vi "CRYGet Selected Rows.vi"(10 "Right Clicked Row":i32=-1, 11 "Tree Ref In":refnum<vi>) -> (3 "Selected Rows":i32[](array[numeric]))   [LabVIEW 2013]
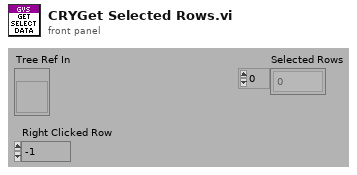
[diagram p1: front panel]
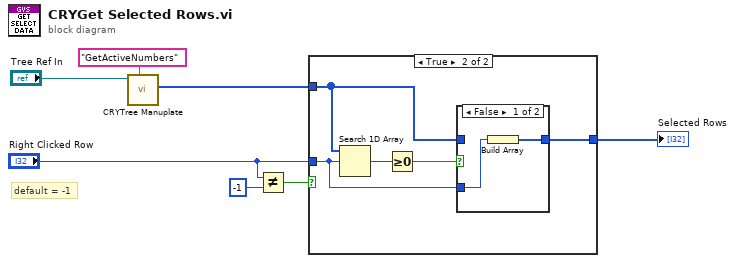
[diagram p0: block diagram]
diagram:
  # "default = -1"
  n1 = call "CRYTree Manuplate.vi"("sAction"="GetActiveNumbers", "Tree in"="Tree Ref In") -> ("nData Out"=w1:i32[])  [unwired: 6 in, 3 out]
  n2 = Not Equal?(x="Right Clicked Row", y=-1) -> (x != y?=w5:bool)
  n3 = case shown="True" w5 {
    tunnel: [w8 w12] -> w7
    tunnel: w1 -> [w8 w11]
    tunnel: "Right Clicked Row" -> [_ w9]
    frame False {
    }
    frame True {
      n4 = Search 1D Array(1D array=w11, element=w9) -> (index of element=w13:i32)  [unwired: 1 out]
      n5 = Greater Or Equal To 0?(x=w13) -> (x >= 0?=w10:bool)
      n6 = case shown="False" w10 {
        tunnel: [w14 w16] -> w12
        tunnel: w11 -> [_ w16]
        tunnel: w9 -> [w15 _]
        frame False {
          n7 = Build Array(w15) -> (w14:i32[])
        }
        frame True {
        }
      }
    }
  }
  "Selected Rows" <- w7
